vi "String Array Pick Subset 02.vi"(4 "# of Columns":i32=1, 5 "# of Rows":i32=25, 6 "Start Col":i32=2, 7 "Start Row":i32=2, 8 "Transpose(F)":bool, 11 "String Array":string[][](array[string])) -> (1 "1d Out":string[](array[string]), 3 "2d Output":string[][](array[string]))   [LabVIEW 2020]
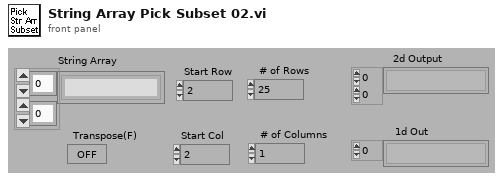
[diagram p1: front panel]
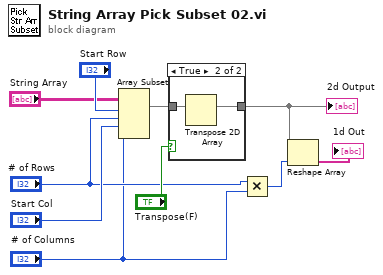
[diagram p0: block diagram]
diagram:
  n1 = Array Subset(array="String Array", index (row)="Start Row", length (row)="# of Rows", index (col)="Start Col", length (col)="# of Columns") -> (w7:string[][])
  n2 = case shown="True" "Transpose(F)" {
    tunnel: w7 -> [w11 w13]
    tunnel: [w11 w12] -> w6
    frame False {
    }
    frame True {
      n3 = Transpose 2D Array(2D array=w13) -> (transposed array=w12:string[][])
    }
  }
  "2d Output" <- w6
  n4 = Multiply(x="# of Rows", y="# of Columns") -> (x*y=w4:i32)
  n5 = Reshape Array(w6, w4) -> (→"1d Out":string[])
